vi "PI_E710_Communicate.vi"(0 "System no.":i32, 2 "String to send":string, 5 "error in":errorcluster) -> (14 "System no. (dup)":i32, 16 "String read":string, 19 "error out":errorcluster)   [LabVIEW 2010]
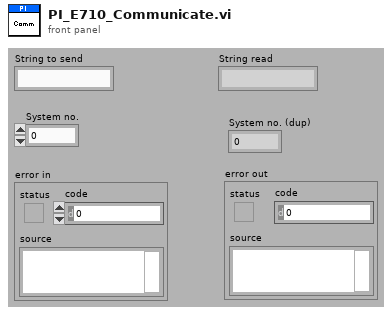
[diagram p1: front panel]
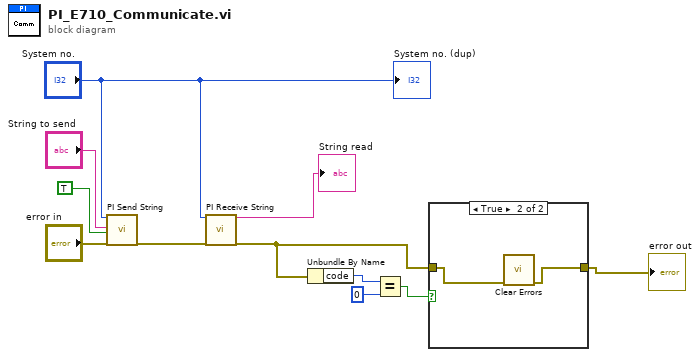
[diagram p0: block diagram]
diagram:
  n1 = call <userlib>:"PI Send String.vi"("System no."="System no.", "String to send"="String to send", "Attach Linefeed?"=TRUE, "error in"="error in") -> ("error out"=w8:errorcluster)  [unwired: 15 out]
  n2 = call <userlib>:"PI Receive String.vi"("System no."="System no.", "error in"=w8) -> ("String read"=→"String read":string, "error out"=w3:errorcluster)  [unwired: 16 out]
  n3 = Unbundle By Name(w3) -> ("code"=w6:i32)
  n4 = Equal?(x=w6, y=0) -> (x = y?=w4:bool)
  n5 = case shown="True" w4 {
    tunnel: w3 -> [w12 w14]
    tunnel: [w12 w13] -> w2
    frame False {
    }
    frame True {
      n6 = call <vilib>:"Clear Errors.vi"("error in (no error)"=w14) -> ("error out"=w13:errorcluster)  [unwired: 6 in]
    }
  }
  "error out" <- w2
  "System no. (dup)" <- "System no."
